vi "PRIME Detector Connect.vi"(8 "error in (no error)":errorcluster, 11 "Detector Computer":T2={"Machine"="192.168.121.11", "Password"="rSL!nux23456", "FITS File Path"="", "Port"=44444, "Header Path"="", "Name"=""}) -> (0 "error out":errorcluster, 1 "Status":T1, 2 "Polling Ref":refnum<k5>, 3 "Cmd Ref":refnum<k5>)   [LabVIEW 2021, in "PRIME Detector.lvclass"]
uses:
  PRIME Detector.lvclass
  RIMAS Detector Server Config.ctl
  PRIME Detector cluster Status.ctl
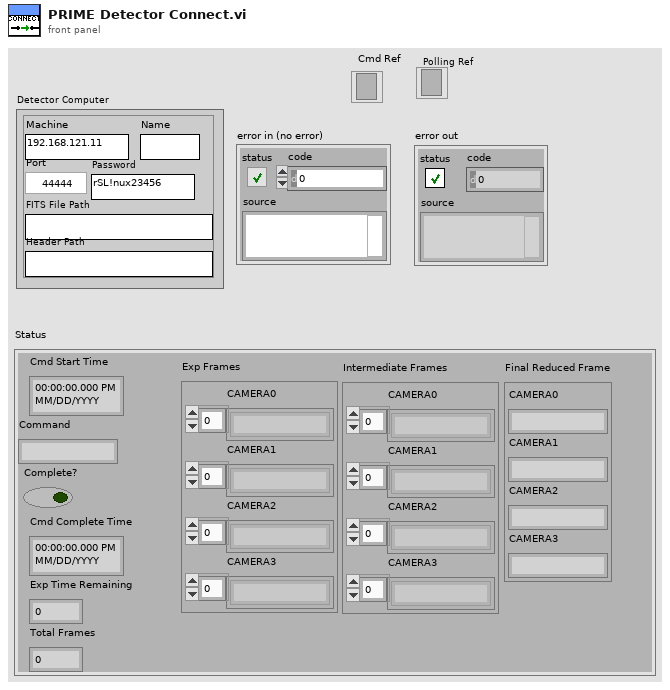
[diagram p1: front panel]
types:
  T1 = typedef "PRIME Detector cluster Status.ctl" = cluster{"Cmd Start Time":timestamp, "Command":string, "Complete?":bool, "Cmd Complete Time":timestamp, "Exp Time Remaining":dbl, "Total Frames":i32, "Exp Frames":cluster{"CAMERA0":string[], "CAMERA1":string[], "CAMERA2":string[], "CAMERA3":string[]}, "Intermediate Frames":cluster{"CAMERA0":string[], "CAMERA1":string[], "CAMERA2":string[], "CAMERA3":string[]}, "Final Reduced Frame":cluster{"CAMERA0":string, "CAMERA1":string, "CAMERA2":string, "CAMERA3":string}}
  T2 = typedef "RIMAS Detector Server Config.ctl" = cluster{"Machine":string, "Password":string, "FITS File Path":string, "Port":u16, "Header Path":string, "Name":string}
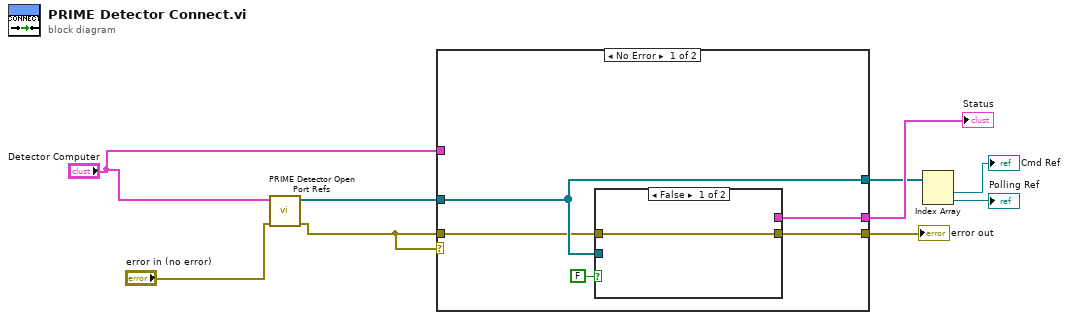
[diagram p0: block diagram]
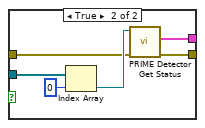
[diagram p2: hidden frame]
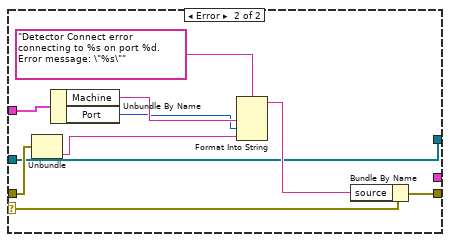
[diagram p3: hidden frame]
diagram:
  n1 = call "PRIME Detector Open Port Refs.vi"("error in (no error)"="error in (no error)", "Settings"="Detector Computer") -> ("error out"=w6:errorcluster, "Connect Refs"=w5:refnum<k5>[])  [unwired: 8 in]
  n2 = case shown="No Error" w6 {
    selector: w6 -> [_ w28]
    tunnel: w6 -> [w11 w30]
    tunnel: w5 -> [w12 w25]
    tunnel: [w14 _] -> w9
    tunnel: [w12 w25] -> w4
    tunnel: [w13 w26] -> w8
    tunnel: "Detector Computer" -> [_ w24]
    frame No Error {
      n3 = case shown="False" FALSE {
        tunnel: [_ w21] -> w14
        tunnel: [w15 w20] -> w13
        tunnel: w12 -> [_ w17]
        tunnel: w11 -> [w15 w16]
        frame False {
        }
        frame True {
          n4 = Index Array(array=w17, index=0) -> (element=w18:refnum<k5>)
          n5 = call "PRIME Detector Get Status.vi"("error in (no error)"=w16, "connection ID"=w18) -> ("error out"=w20:errorcluster, "Status"=w21:T1)  [unwired: 6 in, 2 out]
        }
      }
    }
    frame Error {
      n6 = Unbundle(w30) -> ("source"=w29:string)  [unwired: 2 out]
      n7 = Unbundle By Name(w24) -> ("Machine"=w23:string, "Port"=w22:u16)
      n8 = Format Into String(format string="Detector Connect error connecting to %s on port %d. Error message: \"%s\"", w23, w22, w29) -> (resulting string=w27:string)  [unwired: 2 in, 1 out]
      n9 = Bundle By Name(cluster=w28, "source"=w27) -> (w26:errorcluster)
    }
  }
  "Status" <- w9
  "error out" <- w8
  n10 = Index Array(array=w4) -> (element #1=→"Cmd Ref":refnum<k5>, element #2=→"Polling Ref":refnum<k5>)  [unwired: 2 in]
